vi "RT Device List.vi"(7 "error in (no error)":errorcluster, 10 "Enum":enum16{"Read", "Write"}(ring)) -> (0 "error out":errorcluster, 3 "Channel List":T1)   [LabVIEW 2022 SP3]
uses:
  <resource>/objmgr/daqmx.rc
  64abb6d1-41ad-48eb-9531-31749619ea83.vi
  5481af11-c9d2-47fe-9575-11b741bbd125.vi
  80f775e4-260d-4c3c-b5e2-12464c909832.vi
  4afea8b4-5337-4fb4-93d3-eee184356436.vi
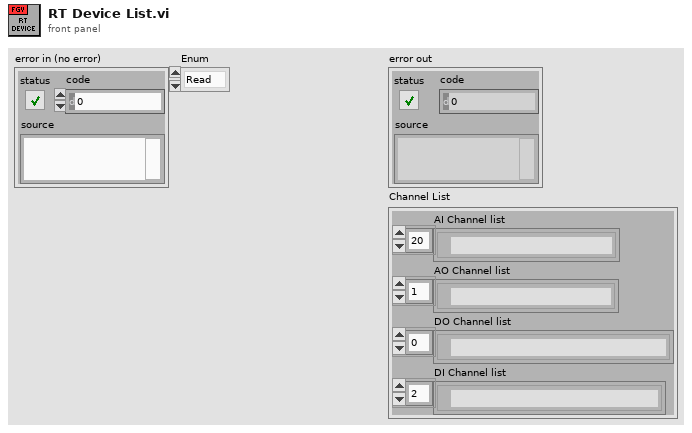
[diagram p1: front panel]
types:
  T1 = cluster{"AI Channel list":tag[], "AO Channel list":tag[], "DO Channel list ":tag[], "DI Channel list":tag[]}
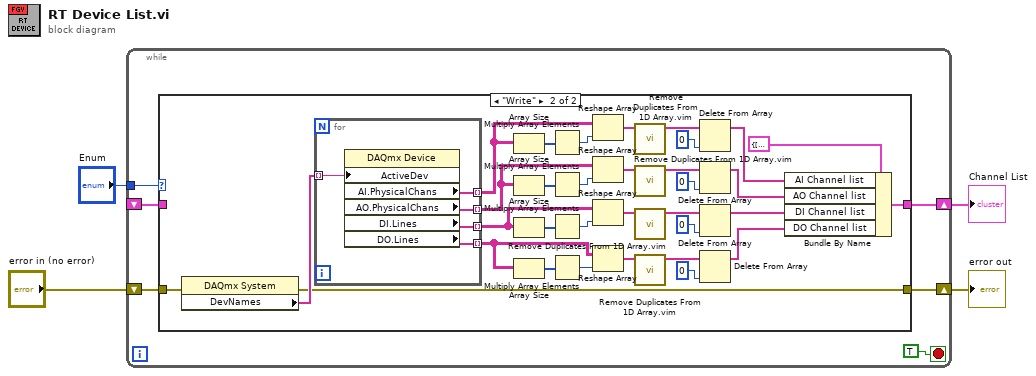
[diagram p0: block diagram]
diagram:
  n1 = while {
    shift-right: [w9] -> w3
    shift-left: "error in (no error)" -> [w10]
    tunnel: "Enum" -> [w7]
    shift-right: [w8] -> w2
    shift-left: _ -> [w6]
    stop <- TRUE stop-if-true
    n2 = case shown="\"Write\"" w7 {
      tunnel: w10 -> [w11 w20]
      tunnel: [w11 w19] -> w9
      tunnel: [w12 w14] -> w8
      tunnel: w6 -> [w12 _]
      frame "Read", Default {
      }
      frame "Write" {
        n3 = property class="DAQmx System"(error in=w20) -> (error out=w19:errorcluster, "DevNames"=w45:tag[])  [unwired: 1 in, 1 out]
        n4 = for {
          tunnel: w45 -> [w48] mode=indexing
          tunnel: [w50] -> w40 mode=indexing
          tunnel: [w49] -> w35 mode=indexing
          tunnel: [w47] -> w26 mode=indexing
          tunnel: [w46] -> w25 mode=indexing
          n5 = property class="DAQmx Device"("ActiveDev"=w48) -> ("AI.PhysicalChans"=w50:tag[], "AO.PhysicalChans"=w49:tag[], "DI.Lines"=w47:tag[], "DO.Lines"=w46:tag[])  [unwired: 2 in, 2 out]
        }
        n6 = Array Size(array=w40) -> (size(s)=w44:i32[])
        n7 = Array Size(array=w35) -> (size(s)=w39:i32[])
        n8 = Array Size(array=w26) -> (size(s)=w34:i32[])
        n9 = Array Size(array=w25) -> (size(s)=w30:i32[])
        n10 = Multiply Array Elements(1:w44) -> (0:w43:i32)
        n11 = Multiply Array Elements(1:w39) -> (0:w38:i32)
        n12 = Multiply Array Elements(1:w34) -> (0:w33:i32)
        n13 = Multiply Array Elements(1:w30) -> (0:w29:i32)
        n14 = Reshape Array(w40, w43) -> (w42:tag[])
        n15 = Reshape Array(w35, w38) -> (w37:tag[])
        n16 = Reshape Array(w26, w33) -> (w32:tag[])
        n17 = Reshape Array(w25, w29) -> (w28:tag[])
        n18 = call "Remove Duplicates From 1D Array.vim"("array"=w42) -> ("array with duplicates removed"=w41:tag[])  [unwired: 10 in]
        n19 = call "Remove Duplicates From 1D Array.vim"("array"=w37) -> ("array with duplicates removed"=w36:tag[])  [unwired: 10 in]
        n20 = call "Remove Duplicates From 1D Array.vim"("array"=w32) -> ("array with duplicates removed"=w31:tag[])  [unwired: 10 in]
        n21 = call "Remove Duplicates From 1D Array.vim"("array"=w28) -> ("array with duplicates removed"=w27:tag[])  [unwired: 10 in]
        n22 = Delete From Array(array=w41, index=0) -> (array with subset deleted=w13:tag[])  [unwired: 1 in, 1 out]
        n23 = Delete From Array(array=w36, index=0) -> (array with subset deleted=w17:tag[])  [unwired: 1 in, 1 out]
        n24 = Delete From Array(array=w31, index=0) -> (array with subset deleted=w16:tag[])  [unwired: 1 in, 1 out]
        n25 = Delete From Array(array=w27, index=0) -> (array with subset deleted=w15:tag[])  [unwired: 1 in, 1 out]
        n26 = Bundle By Name(cluster=T1 {"AI Channel list"=[], "AO Channel list"=[], "DO Channel list "=[], "DI Channel list"=[]} ("Cluster"), "AI Channel list"=w13, "AO Channel list"=w17, "DI Channel list"=w16, "DO Channel list"=w15) -> (w14:T1)
      }
    }
  }
  "error out" <- w3
  "Channel List" <- w2
